vi "GenerateChangedFilesList.vi"(6 "GUI Mode? {F)":bool, 7 "Output File Path":path=path "E:/sw-deps-monitor/changed-files.txt", 8 "error in (no error)":errorcluster, 9 "Branch 2":string="initial-ci-check-yml", 10 "Branch 1":string="main", 11 "Workspace Path":path=path "E:/sw-deps-monitor") -> (0 "error out":errorcluster)   [LabVIEW 2019, in "DepsWatch.lvlib"]
uses:
  DepsWatch.lvlib
  <vilib>/Hampel Software Engineering/Git API/Git API/GIT-api.lvclass/GIT-api.ctl
  <vilib>/Hampel Software Engineering/Git API/Git API/Accessors/GIT-Set Working Dir.vi
  <vilib>/Wiresmith Technology/G CLI/CLI Class/CLI.lvclass
  <vilib>/Hampel Software Engineering/Git API/Git API/GIT-api.lvclass
panel:
  out "std out":string
  in  "Tab Control":T1(tab)
  out "Args":string[](array[string])=["E:\\sw-deps-monitor", "main", "initial-ci-check-yml", "E:\\sw-deps-monitor\\changed-files.txt"]
  # "When in GUI Mode, the controls will be used, \nin CLI Mode the Args will be used"
  # "Workspace Path"
  # "Branch 1"
  # "Branch 2"
  # "Output File Path"
  # "Command to run the VI from terminal\n\ng-cli -v --lv-ver 2023 --arch 32 \"E:\\sw-deps-monitor\\CICD\\Reusables\\GenerateChangedFilesList.vi\" \n-- \"E:\\sw-deps-monitor\" \"main\" \"initial-ci-check-yml\" \"E:\\sw-deps-monitor\\changed-files.txt\""
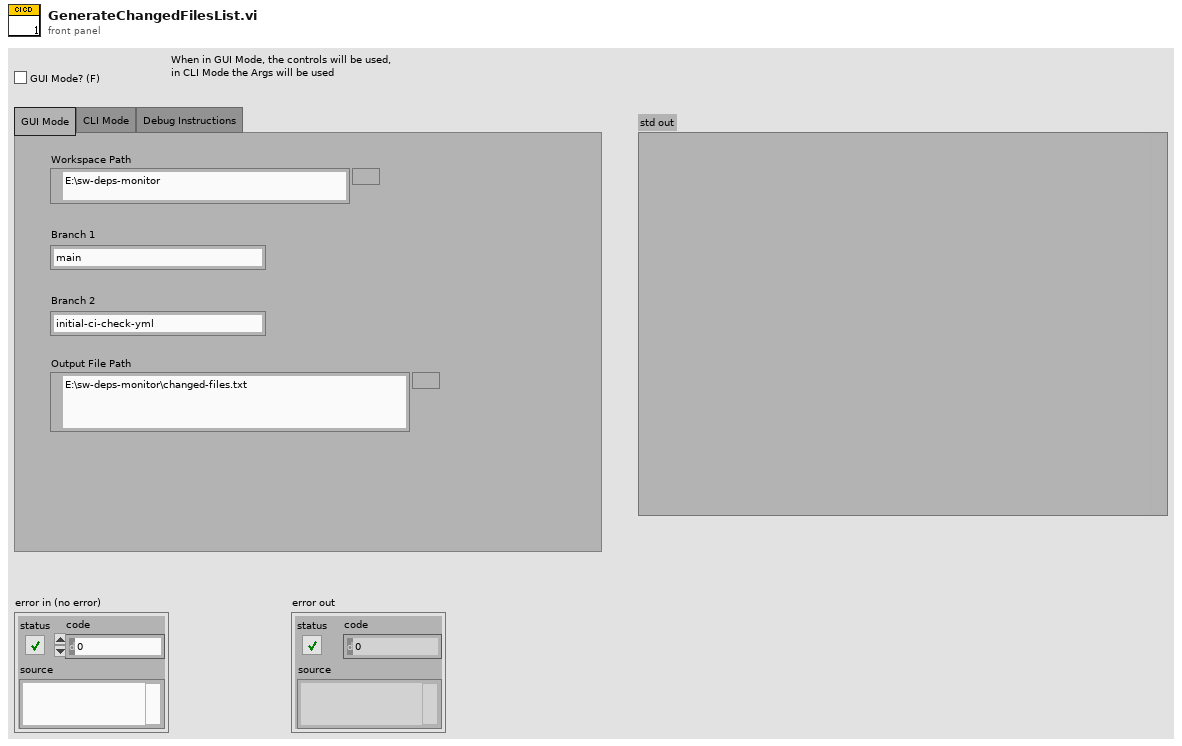
[diagram p1: front panel]
types:
  T1 = enum32{"GUI Mode", "CLI Mode", "Debug Instructions"}
  T2 = enum16{"open", "replace", "create", "open or create", "replace or create", "replace or create with confirmation"}
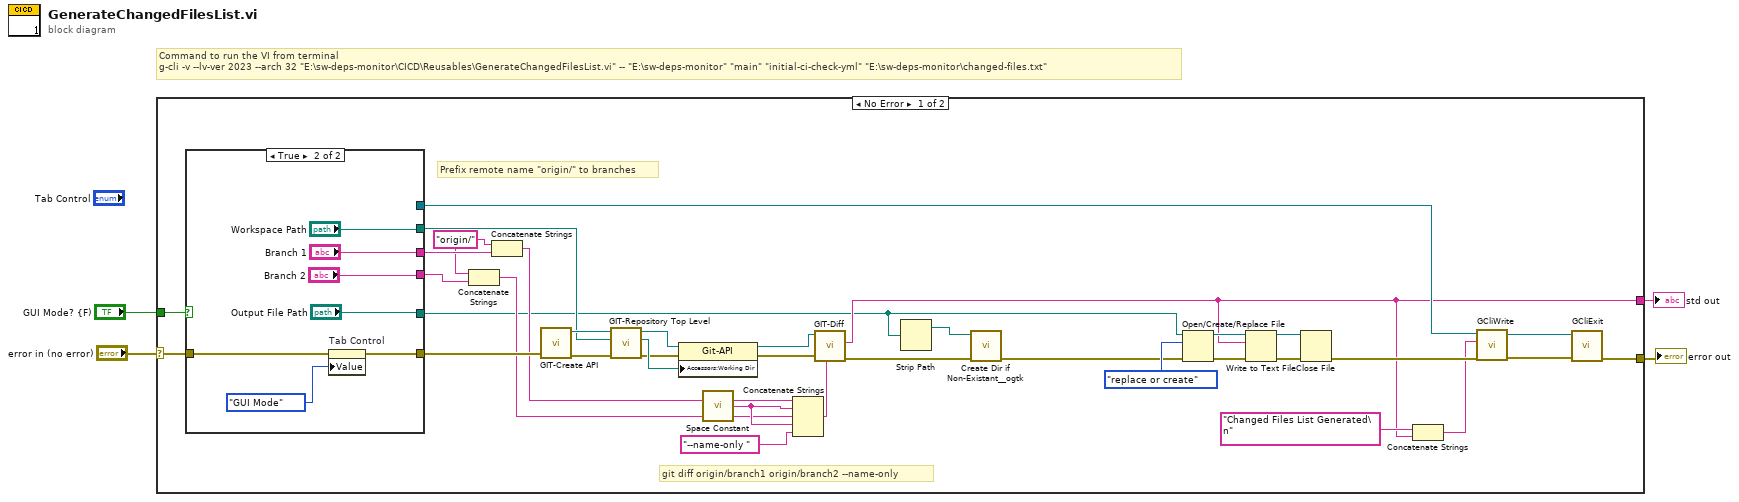
[diagram p0: block diagram]
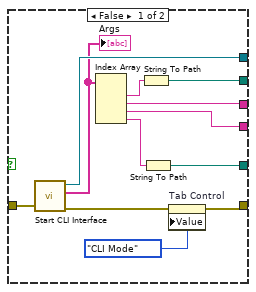
[diagram p2: hidden frame]
diagram:
  # "Command to run the VI from terminal\ng-cli -v --lv-ver 2023 --arch 32 \"E:\\sw-deps-monitor\\CICD\\Reusables\\GenerateChangedFilesList.vi\" -- \"E:\\sw-deps-monitor\" \"main\" \"initial-ci-check-yml\" \"E:\\sw-deps-monitor\\changed-files.txt\""
  n1 = case shown="No Error" "error in (no error)" {
    selector: "error in (no error)" -> [w30 w60]
    tunnel: "GUI Mode? {F)" -> [w31 _]
    tunnel: [w15 _] -> w2
    tunnel: [w18 w60] -> w1
    frame No Error {
      w11 = "origin/" ("string")
      # "git diff origin/branch1 origin/branch2 --name-only"
      # "Prefix remote name \"origin/\" to branches"
      n2 = case shown="True" w31 {
        tunnel: [w51 "Branch 1"] -> w13
        tunnel: [w48 "Workspace Path"] -> w28
        tunnel: [w47 "Output File Path"] -> w8
        tunnel: [w50 "Branch 2"] -> w10
        tunnel: w30 -> [w46 w55]
        tunnel: [w44 w53] -> w29
        tunnel: [w45 _] -> w20
        frame False {
          n3 = call <vilib>:"Start CLI Interface.vi"("error in (no error)"=w46) -> ("error out"=w42:errorcluster, "Custom Parameters"=w41:string[], "CLI out"=w45:refnum<class "CLI.lvclass">)  [unwired: 7 in, 1 out]
          "Args" <- w41
          n4 = Index Array(array=w41) -> (element #1=w52:string, element #2=w51:string, element #3=w50:string, element #4=w49:string)  [unwired: 4 in]
          n5 = String To Path(string=w52) -> (path=w48:path)
          n6 = String To Path(string=w49) -> (path=w47:path)
          n7 = property on="Tab Control" class="TabCtl (strict)"(error in=w42, "Value"=enum32{"GUI Mode", "CLI Mode"}."CLI Mode" ("Tab Control")) -> (error out=w44:errorcluster)  [unwired: 1 in, 1 out]
        }
        frame True {
          n8 = property on="Tab Control" class="TabCtl (strict)"(error in=w55, "Value"=enum32{"GUI Mode", "CLI Mode"}."GUI Mode" ("Tab Control")) -> (error out=w53:errorcluster)  [unwired: 1 in, 1 out]
        }
      }
      n9 = Concatenate Strings(w11, w10) -> (w9:string)
      n10 = Concatenate Strings(w11, w13) -> (w12:string)
      n11 = call <vilib>:"GIT-Create API.vi"("error in"=w29) -> ("error out"=w36:errorcluster, "git-api out"=w39:refnum<class "GIT-api.lvclass">)  [unwired: 9 in]
      n12 = call <vilib>:"GIT-Repository Top Level.vi"("error in"=w36, "Current Path"=w28, "git-api in"=w39) -> ("error out"=w37:errorcluster, "Repo Top Level Path"=w38:path, "git-api out"=w40:refnum<class "GIT-api.lvclass">)  [unwired: 6 in]
      n13 = property class="Git-API"(reference=w40, error in=w37, "Accessors:Working Dir"=w38) -> (reference out=w34:refnum<class "GIT-api.lvclass">, error out=w35:errorcluster)
      n14 = call <vilib>:"Space Constant.vi"() -> ("String"=w27:string)
      n15 = Concatenate Strings(w12, w27, w9, w27, "--name-only " ("string")) -> (w33:string)
      n16 = call <vilib>:"GIT-Diff.vi"("param"=w33, "error in"=w35, "git-api in"=w34) -> ("error out"=w6:errorcluster, "std out"=w15:string)  [unwired: 6 in, 1 out]
      n17 = Strip Path(path=w8) -> (stripped path=w5:path)  [unwired: 1 out]
      n18 = call <userlib>:"Create Dir if Non-Existant__ogtk.vi"("error in (no error)"=w6, "Directory Path"=w5) -> ("error out"=w7:errorcluster)  [unwired: 7 in, 2 out]
      n19 = Open/Create/Replace File(file path (use dialog)=w8, error in=w7, operation (0:open)=T2."replace or create") -> (refnum out=w24:refnum<file>, error out=w25:errorcluster)  [unwired: 3 in, 1 out]
      n20 = Write to Text File(file (use dialog)=w24, text=w15, error in=w25) -> (refnum out=w22:refnum<file>, error out=w23:errorcluster)  [unwired: 1 in, 1 out]
      n21 = Close File(refnum=w22, error in=w23) -> (error out=w21:errorcluster)  [unwired: 1 out]
      n22 = Concatenate Strings("Changed Files List Generated\n" ("Text to Write"), w15) -> (w14:string)
      n23 = call "GCliWrite.vi"("error in (no error)"=w21, "Text to Write"=w14, "CLI in"=w20) -> ("error out"=w19:errorcluster, "CLI out"=w17:refnum<class "CLI.lvclass">)  [unwired: 7 in]
      n24 = call "GCliExit.vi"("error in (no error)"=w19, "CLI in"=w17) -> ("error out"=w18:errorcluster)  [unwired: 9 in]
    }
    frame Error {
    }
  }
  "error out" <- w1
  "std out" <- w2
